vi "getInput.vi"(8 "error in (no error)":errorcluster, 11 "PrettyPrinting.lvclass in":refnum<class "PrettyPrinting.lvclass">) -> (0 "error out":errorcluster, 2 "input":string, 3 "PrettyPrinting.lvclass out":refnum<class "PrettyPrinting.lvclass">)   [LabVIEW 2011, in "Views.lvlib" / "ViewerTools.lvlib" / "PrettyPrinting.lvclass"]
uses:
  PrettyPrinting.lvclass
  PrettyPrinting.lvclass/PrettyPrinting.ctl
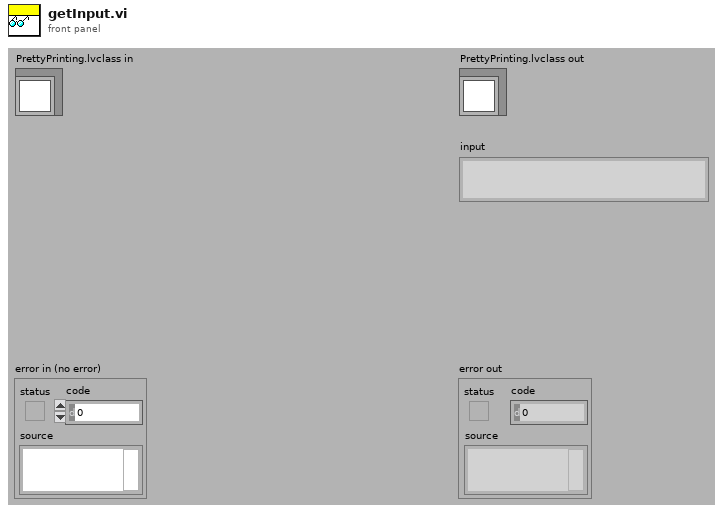
[diagram p1: front panel]
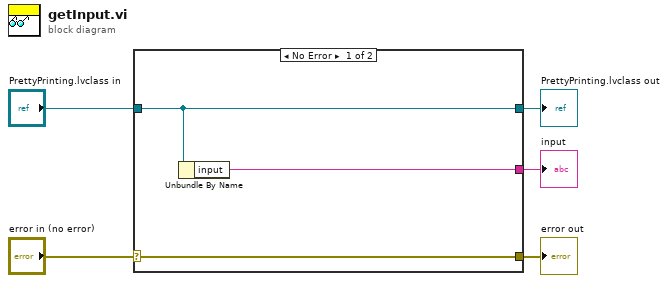
[diagram p0: block diagram]
diagram:
  n1 = case shown="No Error" "error in (no error)" {
    selector: "error in (no error)" -> [w8 w9]
    tunnel: [w8 w9] -> w4
    tunnel: [w7 w10] -> w2
    tunnel: "PrettyPrinting.lvclass in" -> [w7 w10]
    tunnel: [w6 _] -> w1
    frame No Error {
      n2 = Unbundle By Name(w7) -> ("input"=w6:string)
    }
    frame Error {
    }
  }
  "error out" <- w4
  "PrettyPrinting.lvclass out" <- w2
  "input" <- w1
